vi "Get Coordinates.vi"(8 "error in (no error)":errorcluster, 9 "Plot ID":i32, 11 "3D Comet.lvclass in":refnum<class "3D Comet.lvclass">) -> (0 "error out":errorcluster, 1 "Coordinates System":enum16{"Cartesian", "Cylindrical", "Spherical"}(ring), 3 "3D Comet.lvclass out":refnum<class "3D Comet.lvclass">)   [LabVIEW 2017, in "3D Comet.lvclass"]
uses:
  <vilib>/Math Plots/3D Math Plots/3D Comet/3D Comet/3D Comet.lvclass
  <vilib>/Math Plots/3D Math Plots/3D Comet/3D Comet/3D Comet.lvclass/3D Comet.ctl
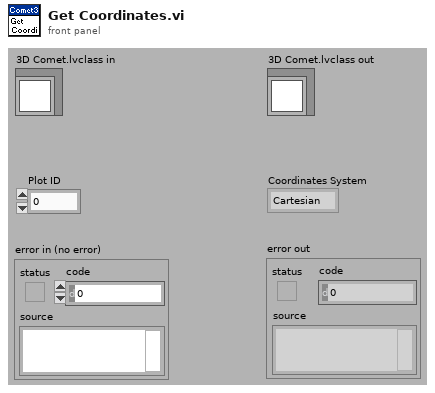
[diagram p1: front panel]
types:
  T1 = typedef "3D Comet.lvclass/3D Comet Property Array.ctl" = T2[]
  T2 = typedef "3D Comet.lvclass/3D Comet Property.ctl" = cluster{"General Property":cluster{"Plot Name":string, "Coordinate System":enum16{"Cartesian", "Cylindrical", "Spherical"}, "Opacity":sgl}, "Projection Property":cluster{"Draw XY":bool, "Draw YZ":bool, "Draw XZ":bool}, "Plot Property":cluster{"Sprite Type":T3, "Point Size":sgl, "Point Color":u32, "Line Style":T4, "Line Width":sgl, "Line Color":u32, "Antialiasing":bool}, "Comet Property":cluster{"Body length":sgl}}
  T3 = typedef "3D Plot.lvclass/Sprite Type.ctl" = enum16{"None", "Empty Square", "Solid Square", "Empty Diamond", "Solid Diamond", "Empty Circle", "Solid Circle", "Asterisk", "Bold X", "Wireframe Sphere", "Solid Sphere", "Wireframe Cube", "Solid Cube"}
  T4 = typedef "3D Plot.lvclass/Line Type.ctl" = enum16{"None", "Solid", "Dash", "Dot", "Dash Dot"}
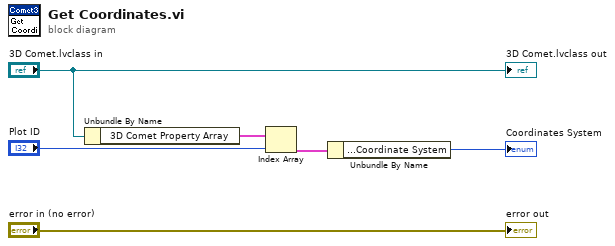
[diagram p0: block diagram]
diagram:
  n1 = Unbundle By Name("3D Comet.lvclass in") -> ("3D Comet Property Array"=w6:T1)
  n2 = Index Array(array=w6, index="Plot ID") -> (element=w5:T2)
  n3 = Unbundle By Name(w5) -> ("General Property.Coordinate System"=→"Coordinates System":enum16{"Cartesian", "Cylindrical", "Spherical"})
  "3D Comet.lvclass out" <- "3D Comet.lvclass in"
  "error out" <- "error in (no error)"
